vi "Launch Aggregate Model (Explicit).vi"(8 "error in (no error)":errorcluster, 10 "Model to Launch":refnum<class "IModel.lvclass">, 11 "IModel in":refnum<class "IModel.lvclass">) -> (0 "error out":errorcluster, 2 "Nested Model's Enqueuer":refnum<class "Message Enqueuer.lvclass">, 3 "IModel out":refnum<class "IModel.lvclass">)   [LabVIEW 2017, in "IModel.lvlib" / "IModel.lvclass"]
uses:
  IModel.lvclass
  C:/Program Files (x86)/National Instruments/LabVIEW 2017/vi.lib/ActorFramework/Actor/Actor.lvclass
  C:/Git/mva-framework/Source/Framework/IObserver/IObserver/IObserver.lvclass
  <vilib>/ActorFramework/Message Enqueuer/Message Enqueuer.lvclass
  IObserver/IObserver/IObserver.lvclass/IObserver.ctl
  IModel.lvclass/IModel.ctl
  IObserver/IObserver/Read Subscribe Msg.vi
  IObserver/IObserver/Read Unsubscribe Msg.vi
  IObserver/IObserver/Write Pre-Addressed Observer Msgs.vi
  <vilib>/ActorFramework/Actor/Actor.lvclass
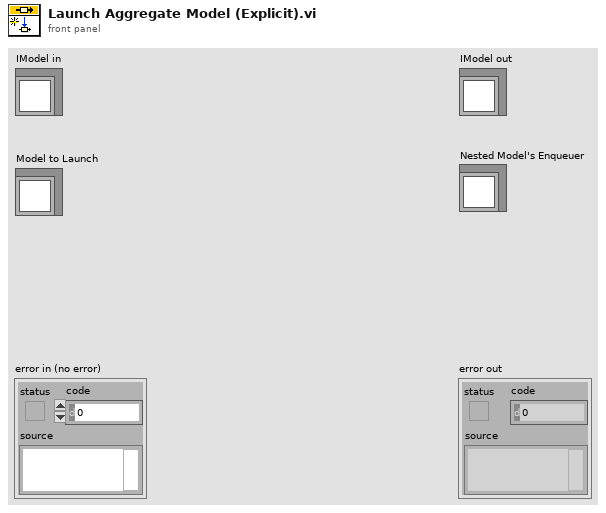
[diagram p1: front panel]
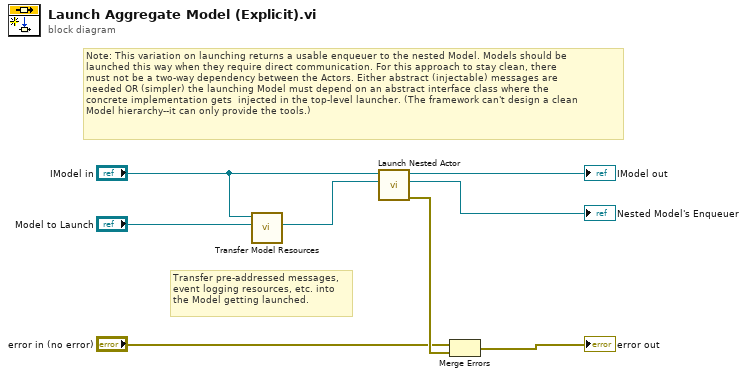
[diagram p0: block diagram]
diagram:
  # "Transfer pre-addressed messages,\nevent logging resources, etc. into\nthe Model getting launched."
  # "Note: This variation on launching returns a usable enqueuer to the nested Model. Models should be\nlaunched this way when they require direct communication. For this approach to stay clean, there\nmust not be a two-way dependency between the Actors. Either abstract (injectable) messages are\nneeded OR (simpler) the launching Model must depend on an abstract interface class where the\nconcrete implementation gets  injected in the top-level launcher. (The framework can't design a clean\nModel hierarchy--it can only provide the tools.)"
  n1 = call "Transfer Model Resources.vi"("Recipient Model In"="Model to Launch", "Launcher Model"="IModel in") -> ("Recipient Model Out"=w1:refnum<class "IModel.lvclass">)  [unwired: 9 in]
  n2 = call <vilib>:"Launch Nested Actor.vi"("Nested Actor"=w1, "Caller Actor in"="IModel in") -> ("error out"=w6:errorcluster, "Nested Actor's Enqueuer"=→"Nested Model's Enqueuer":refnum<class "Message Enqueuer.lvclass">, "Caller Actor out"=→"IModel out":refnum<class "IModel.lvclass">)  [unwired: 7 in]
  n3 = Merge Errors("error in (no error)", w6) -> (→"error out":errorcluster)
